vi "Super Market Billing System edit 3.3.vi"() -> ()   [LabVIEW 2021]
uses:
  <vilib>/Utility/file.llb/Write Delimited Spreadsheet (DBL).vi
  <vilib>/regexp/Match Regular Expression.xnode
panel:
  in  "Tab Control":enum32{"Page 1", "Page 2"}(tab)
  in  "file path (dialog if empty) 2":path
  out "Horizontal Progress Bar":u8(slide) scale=0.0..100.0
  in  "String 2":string
  in  "String":string
  in  "OK Button":bool
  in  "stop":bool
  in  "Rise 5Kg":bool
  in  "Dal 1Kg":bool
  in  "Salt 400g":bool
  in  "Coconut Oil 1L":bool
  in  "Cilli Powder 100g":bool
  in  "Curry Powder 100g":bool
  in  "Turmeric Powder 50g":bool
  in  "Milk Powder 1kg":bool
  in  "Sugar  1kg":bool
  out "Rs.":dbl
  out "Rs.":dbl
  out "Rs.":dbl
  out "Rs.":dbl
  in  "quantity 14":dbl
  out "Rs.":dbl
  in  "quantity 15":dbl
  out "Rs":dbl
  in  "quantity 16":dbl
  out "Rs.":dbl
  in  "quantity 13":dbl
  in  "Quantities 4":dbl
  in  "quantity 12":dbl
  in  "quantity 11":dbl
  in  "quantity 10":dbl
  in  "Tea 100g":bool
  in  "Quantities":dbl
  in  "quantity 17":dbl
  out "Rs.":dbl
  out "Rs.":dbl
  out "Rs.":dbl
  out "Rs.":dbl
  out "Rs.":dbl
  out "Rs.":dbl
  out "Rs.":dbl
  out "Rs. 5":dbl
  out "Rs. 6":dbl
  out "Rs.":dbl
  out "Rs.":dbl
  out "Rs.":dbl
  out "Rs.":dbl
  out "Discount   Rs.":dbl
  in  "kg":dbl
  in  "Papaya":bool
  in  "kg":dbl
  in  "Graps":bool
  in  "kg":dbl
  in  "Orange":bool
  in  "kg":dbl
  in  "Apple":bool
  in  "kg":dbl
  in  "Banana":bool
  out "Bill   Rs.":dbl
  out "Discount percentage":string
  out "Total Bill   Rs.":dbl
  in  "kg":dbl
  in  "Cabege":bool
  in  "kg":dbl
  in  "Bringle":bool
  in  "kg":dbl
  in  "Beans":bool
  in  "kg":dbl
  in  "Leeks":bool
  in  "kg":dbl
  in  "Carrot":bool
  # "WELCOME TO A SUPER MARCKET...."
  # "Price per 1kg (Rs.)"
  # "Quantities(kg)"
  # "Price  (Rs.)"
  # "Quantities"
  # "Vegetables"
  # "Product List"
  # "Fruits"
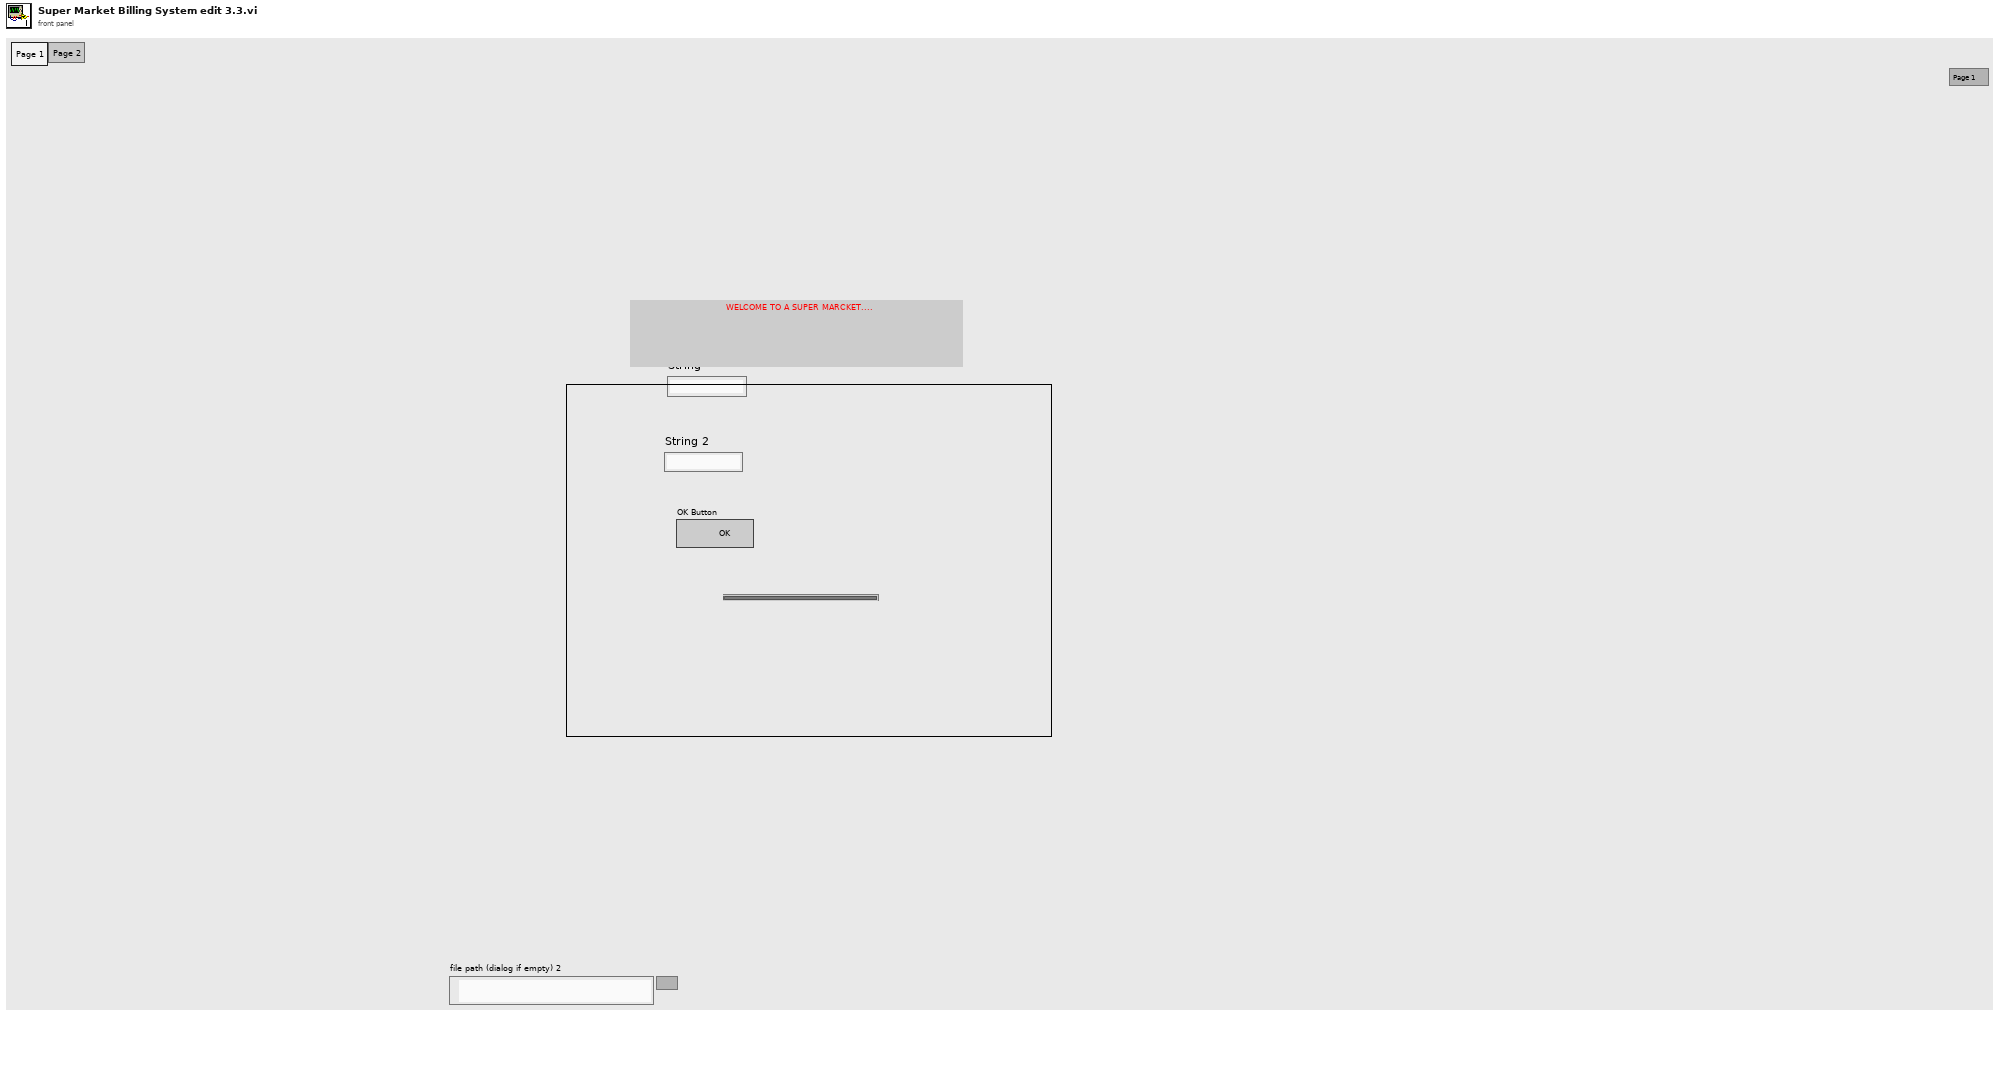
[diagram p1: front panel]
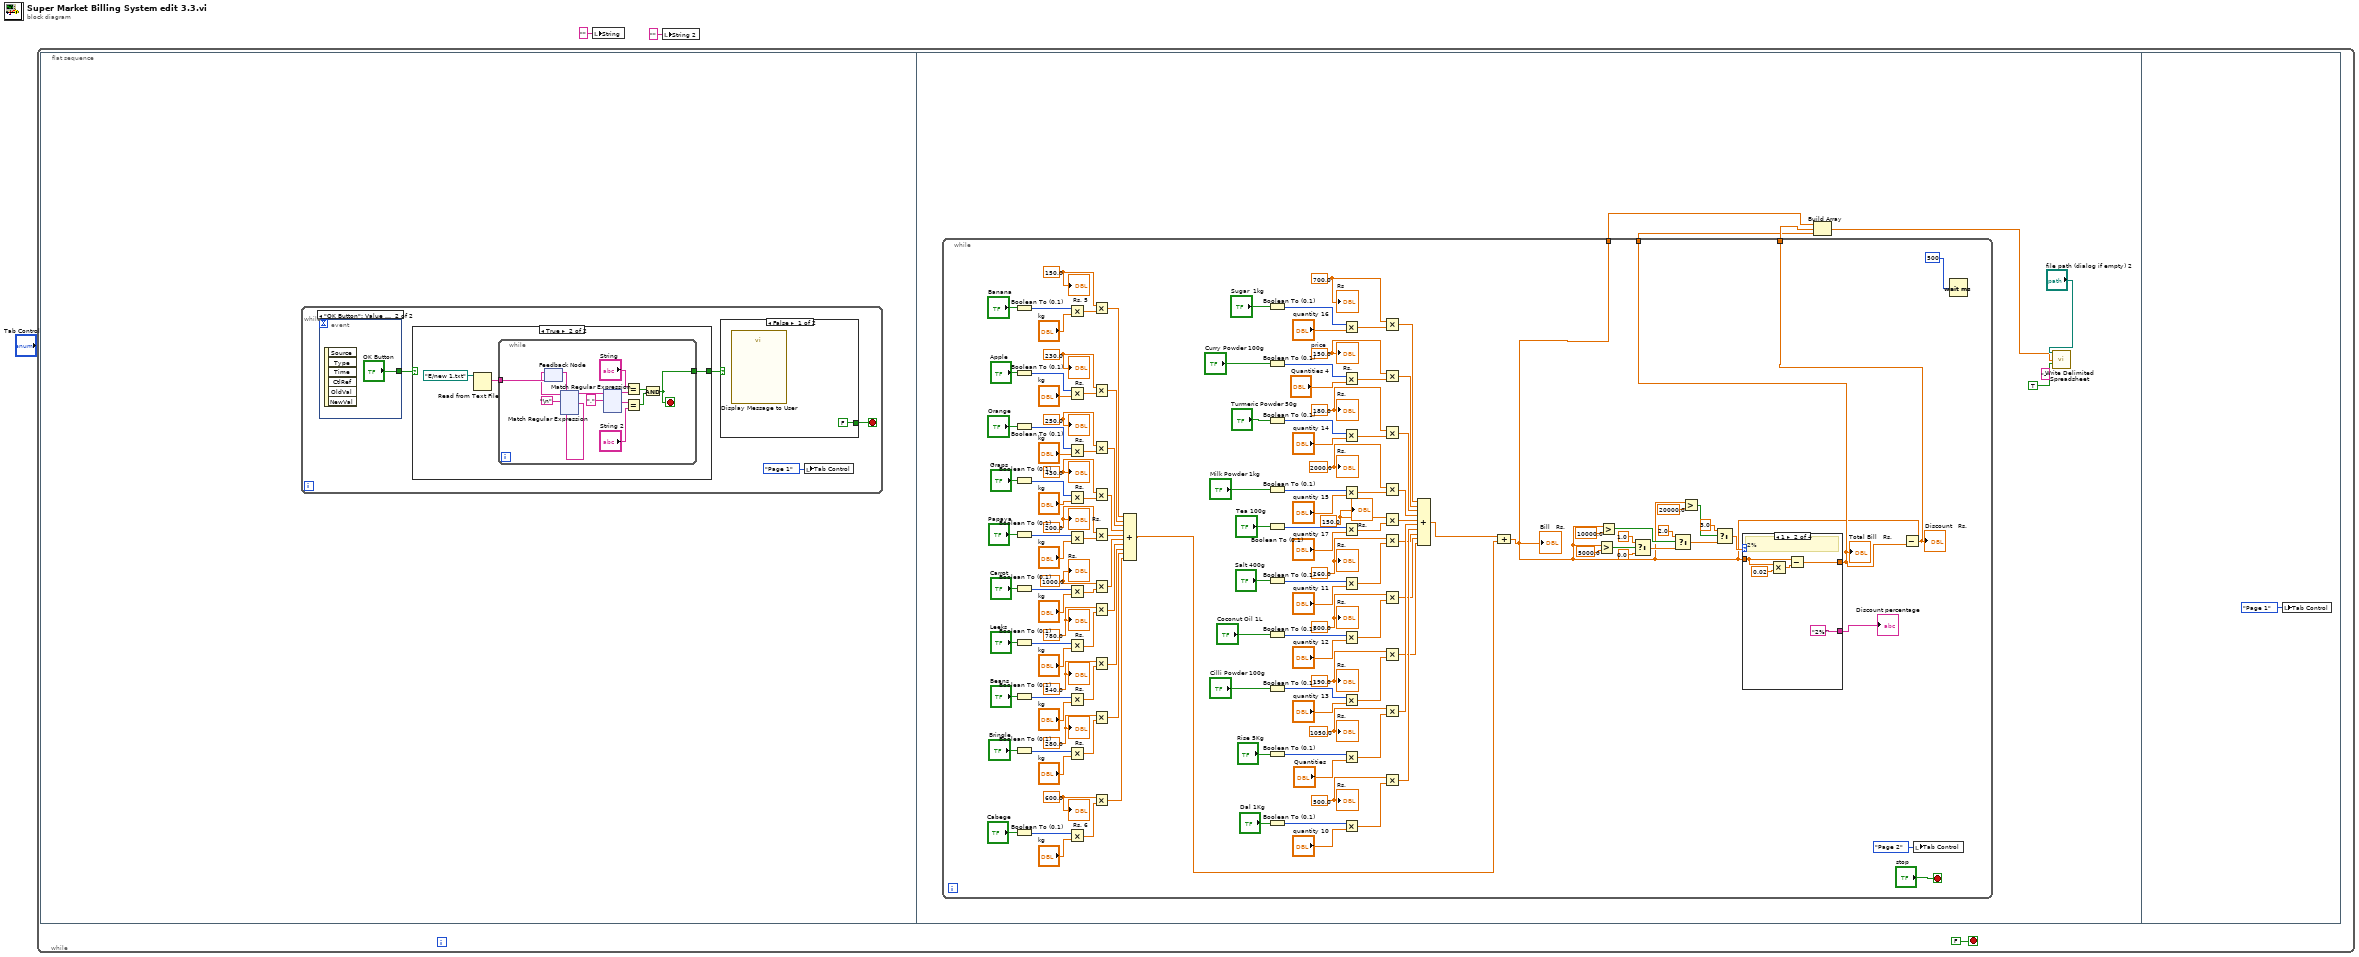
[diagram p0: block diagram]
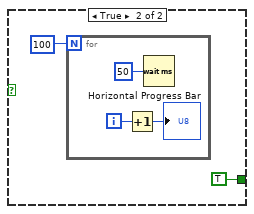
[diagram p2: hidden frame]
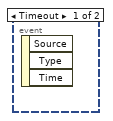
[diagram p4: hidden frame]
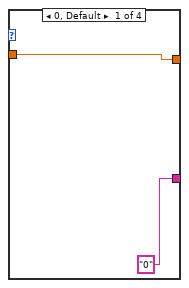
[diagram p5: hidden frame]
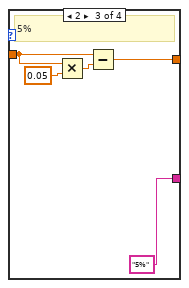
[diagram p6: hidden frame]
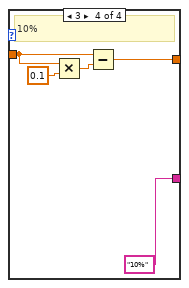
[diagram p7: hidden frame]
diagram:
  n1 = while {
    stop <- FALSE stop-if-true
    n2 = flat-sequence {
      frame #0 {
        n3 = while {
          stop <- w5 stop-if-true
          n4 = event shown="[1] \"OK Button\": Value Change" {
            selector: _ -> [_ _]
            dyn-events: _ -> [_ _]
            timeout: _ -> [_ _]
            tunnel: [_ "OK Button"] -> w7
            event Timeout {
              n5 = event-data() -> ()  [unwired: 1 in, 3 out]
            }
            event "OK Button": Value Change {
              n6 = event-data() -> ()  [unwired: 1 in, 6 out]
            }
          }
          n7 = case shown="True" w7 {
            selector: w7 -> [w14 _]
            tunnel: [w14 w15] -> w6
            frame False {
            }
            frame True {
              n8 = Read from Text File(file (use dialog)=path "E:/new 1.txt") -> (text=w17:string)  [unwired: 3 in, 3 out]
              n9 = while {
                tunnel: w17 -> [w30]
                tunnel: [w18] -> w15
                stop <- w18 stop-if-true
                n10 = feedback #1(w30) -> (w29:string)
                n11 = xnode "Match Regular Expression"("input string"=w29, "regular expression"="\n") -> ("before match"=w26:string, "after match"=w28:string)  [unwired: 4 in, 3 out]
                n12 = feedback-in #1(w28) -> ()
                n13 = xnode "Match Regular Expression"("input string"=w26, "regular expression"=",") -> ("before match"=w23:string, "after match"=w24:string)  [unwired: 4 in, 3 out]
                n14 = Equal?(x="String", y=w23) -> (x = y?=w20:bool)
                n15 = Equal?(x=w24, y="String 2") -> (x = y?=w19:bool)
                n16 = And(x=w20, y=w19) -> (x .and. y?=w18:bool)
              }
            }
          }
          n17 = case shown="False" w6 {
            tunnel: [FALSE TRUE] -> w5
            frame False {
              n18 = call "Display Message to User"() -> ()  [unwired: 10 in, 2 out]
            }
            frame True {
              n19 = for {
                N: 100 -> [_]
                i -> [w11]
                n20 = Increment(x=w11) -> (x+1=→"Horizontal Progress Bar":i32)
                n21 = Wait (ms)(milliseconds to wait=u32 50 ("millisecond timer value")) -> ()  [unwired: 1 out]
              }
            }
          }
          n22 = local write "Tab Control"(enum32{"Page 1", "Page 2"}."Page 1" ("Tab Control")) -> ()
        }
      }
      frame #1 {
        n23 = while {
          tunnel: [w273] -> w272
          tunnel: [w274] -> w266
          tunnel: [w275] -> w267
          stop <- "stop" stop-if-true
          w301 = 200.0 ("price")
          w294 = 430.0 ("price")
          w291 = 250.0 ("price")
          w284 = 230.0 ("price")
          w281 = 150.0 ("price")
          w326 = 600.0 ("price")
          w319 = 280.0 ("price")
          w316 = 540.0 ("price")
          w309 = 780.0 ("price")
          w306 = 1000.0 ("price")
          w387 = 150.0 ("price")
          w380 = 700.0 ("price")
          w377 = 2000.0 ("price")
          w370 = 180.0 ("price")
          w367 = 150.0  # price
          w412 = 190.0 ("price")
          w405 = 800.0 ("price")
          w402 = 260.0 ("price")
          w395 = 500.0 ("price")
          w392 = 1050.0 ("price")
          n24 = Boolean To (0,1)(Boolean="Banana") -> (0, 1=w279:i16)
          n25 = Boolean To (0,1)(Boolean="Apple") -> (0, 1=w286:i16)
          n26 = Boolean To (0,1)(Boolean="Orange") -> (0, 1=w289:i16)
          n27 = Boolean To (0,1)(Boolean="Graps") -> (0, 1=w296:i16)
          n28 = Boolean To (0,1)(Boolean="Papaya") -> (0, 1=w299:i16)
          n29 = Boolean To (0,1)(Boolean="Carrot") -> (0, 1=w304:i16)
          n30 = Boolean To (0,1)(Boolean="Leeks") -> (0, 1=w311:i16)
          n31 = Boolean To (0,1)(Boolean="Beans") -> (0, 1=w314:i16)
          n32 = Boolean To (0,1)(Boolean="Bringle") -> (0, 1=w321:i16)
          n33 = Boolean To (0,1)(Boolean="Cabege") -> (0, 1=w324:i16)
          n34 = Multiply(x=w279, y="kg") -> (x*y=w282:dbl)
          n35 = Multiply(x=w286, y="kg") -> (x*y=w283:dbl)
          n36 = Multiply(x=w289, y="kg") -> (x*y=w292:dbl)
          n37 = Multiply(x=w296, y="kg") -> (x*y=w293:dbl)
          n38 = Multiply(x=w299, y="kg") -> (x*y=w302:dbl)
          n39 = Multiply(x=w304, y="kg") -> (x*y=w307:dbl)
          n40 = Multiply(x=w311, y="kg") -> (x*y=w308:dbl)
          n41 = Multiply(x=w314, y="kg") -> (x*y=w317:dbl)
          n42 = Multiply(x=w321, y="kg") -> (x*y=w318:dbl)
          n43 = Multiply(x=w324, y="kg") -> (x*y=w327:dbl)
          n44 = Multiply(x=w281, y=w282) -> (x*y=w342:dbl)
          n45 = Multiply(x=w284, y=w283) -> (x*y=w343:dbl)
          n46 = Multiply(x=w291, y=w292) -> (x*y=w344:dbl)
          n47 = Multiply(x=w294, y=w293) -> (x*y=w345:dbl)
          n48 = Multiply(x=w301, y=w302) -> (x*y=w346:dbl)
          n49 = Multiply(x=w306, y=w307) -> (x*y=w347:dbl)
          n50 = Multiply(x=w309, y=w308) -> (x*y=w348:dbl)
          n51 = Multiply(x=w316, y=w317) -> (x*y=w349:dbl)
          n52 = Multiply(x=w319, y=w318) -> (x*y=w350:dbl)
          n53 = Multiply(x=w326, y=w327) -> (x*y=w351:dbl)
          n54 = Compound Arithmetic op=ADD(w342, w343, w344, w345, w346, w347, w348, w349, w350, w351) -> (w276:dbl)
          n55 = Boolean To (0,1)(Boolean="Sugar  1kg") -> (0, 1=w382:i16)
          n56 = Boolean To (0,1)(Boolean="Curry Powder 100g") -> (0, 1=w365:i16)
          n57 = Boolean To (0,1)(Boolean="Turmeric Powder 50g") -> (0, 1=w372:i16)
          n58 = Boolean To (0,1)(Boolean="Milk Powder 1kg") -> (0, 1=w375:i16)
          n59 = Boolean To (0,1)(Boolean="Tea 100g") -> (0, 1=w385:i16)
          n60 = Boolean To (0,1)(Boolean="Salt 400g") -> (0, 1=w400:i16)
          n61 = Boolean To (0,1)(Boolean="Coconut Oil 1L") -> (0, 1=w407:i16)
          n62 = Boolean To (0,1)(Boolean="Cilli Powder 100g") -> (0, 1=w410:i16)
          n63 = Boolean To (0,1)(Boolean="Rise 5Kg") -> (0, 1=w390:i16)
          n64 = Boolean To (0,1)(Boolean="Dal 1Kg") -> (0, 1=w397:i16)
          n65 = Multiply(x=w382, y="quantity 16") -> (x*y=w379:dbl)
          n66 = Multiply(x=w365, y="Quantities 4") -> (x*y=w368:dbl)
          n67 = Multiply(x=w372, y="quantity 14") -> (x*y=w369:dbl)
          n68 = Multiply(x=w375, y="quantity 15") -> (x*y=w378:dbl)
          n69 = Multiply(x=w385, y="quantity 17") -> (x*y=w388:dbl)
          n70 = Multiply(x=w400, y="quantity 11") -> (x*y=w403:dbl)
          n71 = Multiply(x=w407, y="quantity 12") -> (x*y=w404:dbl)
          n72 = Multiply(x=w410, y="quantity 13") -> (x*y=w413:dbl)
          n73 = Multiply(x=w390, y="Quantities") -> (x*y=w393:dbl)
          n74 = Multiply(x=w397, y="quantity 10") -> (x*y=w394:dbl)
          n75 = Multiply(x=w380, y=w379) -> (x*y=w352:dbl)
          n76 = Multiply(x=w367, y=w368) -> (x*y=w361:dbl)
          n77 = Multiply(x=w370, y=w369) -> (x*y=w360:dbl)
          n78 = Multiply(x=w377, y=w378) -> (x*y=w359:dbl)
          n79 = Multiply(x=w387, y=w388) -> (x*y=w358:dbl)
          n80 = Multiply(x=w402, y=w403) -> (x*y=w355:dbl)
          n81 = Multiply(x=w405, y=w404) -> (x*y=w354:dbl)
          n82 = Multiply(x=w412, y=w413) -> (x*y=w353:dbl)
          n83 = Multiply(x=w392, y=w393) -> (x*y=w357:dbl)
          n84 = Multiply(x=w395, y=w394) -> (x*y=w356:dbl)
          n85 = Compound Arithmetic op=ADD(w352, w361, w360, w359, w358, w357, w356, w355, w354, w353) -> (w277:dbl)
          n86 = Compound Arithmetic op=ADD(w277, w276) -> (w273:dbl)
          "Bill   Rs." <- w273
          n87 = Greater?(x=w273, y=5000.0) -> (0:w339:bool)
          n88 = Greater?(x=w273, y=10000.0) -> (0:w340:bool)
          n89 = Select(t=1.0, s=w339, f=0.0) -> (s? t:f=w335:dbl)
          n90 = Select(t=2.0, s=w340, f=w335) -> (s? t:f=w336:dbl)
          n91 = Greater?(x=w273, y=20000.0) -> (0:w341:bool)
          n92 = Select(t=3.0, s=w341, f=w336) -> (s? t:f=w337:dbl)
          n93 = case shown="1" w337 {
            tunnel: [w416 w420 w423 w428] -> w274
            tunnel: w273 -> [w416 w419 w424 w429]
            tunnel: ["0" ("discount") "2%" ("discount") "5%" ("discount") "10%" ("discount")] -> w338
            frame 0, Default {
            }
            frame 1 {
              # "2%"
              n94 = Multiply(x=w419, y=0.02) -> (x*y=w417:dbl)
              n95 = Subtract(x=w419, y=w417) -> (x-y=w420:dbl)
            }
            frame 2 {
              # "5%"
              n96 = Multiply(x=w424, y=0.05) -> (x*y=w425:dbl)
              n97 = Subtract(x=w424, y=w425) -> (x-y=w423:dbl)
            }
            frame 3 {
              # "10%"
              n98 = Multiply(x=w429, y=0.1) -> (x*y=w430:dbl)
              n99 = Subtract(x=w429, y=w430) -> (x-y=w428:dbl)
            }
          }
          "Total Bill   Rs." <- w274
          "Discount percentage" <- w338
          n100 = Subtract(x=w273, y=w274) -> (x-y=w275:dbl)
          "Discount   Rs." <- w275
          n101 = local write "Tab Control"(enum32{"Page 1", "Page 2"}."Page 2" ("Tab Control")) -> ()
          n102 = Wait (ms)(milliseconds to wait=u32 500) -> ()  [unwired: 1 out]
          "Rs." <- w392
          "Rs." <- w395
          "Rs." <- w402
          "Rs." <- w405
          "Rs." <- w412
          "Rs." <- w367
          "Rs." <- w370
          "Rs." <- w377
          "Rs" <- w380
          "Rs." <- w387
          "Rs." <- w306
          "Rs." <- w309
          "Rs." <- w316
          "Rs." <- w319
          "Rs. 6" <- w326
          "Rs. 5" <- w281
          "Rs." <- w284
          "Rs." <- w291
          "Rs." <- w294
          "Rs." <- w301
        }
        n103 = Build Array "Build Array"(w272, w267, w266) -> (w270:dbl[])
        n104 = call-poly <vilib>:"Write Delimited Spreadsheet.vi"("file path (dialog if empty)"="file path (dialog if empty) 2", "1D data"=w270, "append to file? (new file:F)"=TRUE, "delimiter (\\t)"="-" ("delimiter (\\t)")) -> ()  [unwired: 10 in, 2 out]
      }
      frame #2 {
        n105 = local write "Tab Control"(enum32{"Page 1", "Page 2"}."Page 1" ("Tab Control")) -> ()
      }
    }
  }
  n106 = local write "String"("" ("String")) -> ()
  n107 = local write "String 2"("" ("String 2")) -> ()
